vi "SQRT.vi"(1 "Number":dbl) -> (0 "Square Root":dbl)   [LabVIEW 2017]
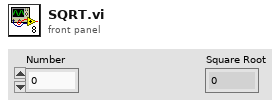
[diagram p1: front panel]
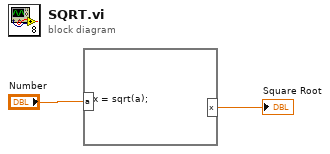
[diagram p0: block diagram]
diagram:
  n1 = formula code="x = sqrt(a);"("a"="Number") -> ("x"=→"Square Root":dbl)
